vi "Server Create Event.vi"(8 "error in":errorcluster, 11 "server event ref":refnum<vi>) -> (0 "error out":errorcluster, 3 "server command event":refnum<user-event>)   [LabVIEW 2013]
doc: "Create user event for server operation commands."
uses:
  Server Event Start.ctl
  measure/Meas Sampling Configuration.ctl
  adc/ADC Trig Config.ctl
  adc/ADC Trig Mode Source.ctl
  adc/ADC Trig Coupling.ctl
  adc/ADC Trig Slope.ctl
  measure/processing/QWTB/Meas Proc QWTB Algorithm Parameter Data.ctl
  measure/processing/Meas Process Mode.ctl
  measure/processing/Meas Process Config.ctl
  measure/processing/Meas Process Raw Config.ctl
  measure/processing/Meas Process Raw Result Mode.ctl
  measure/processing/QWTB/Meas Proc QWTB Setup.ctl
  measure/processing/QWTB/Meas Proc QWTB Uncertainty Mode.ctl
  Server Event GUI command.ctl
  Server Event Command.ctl
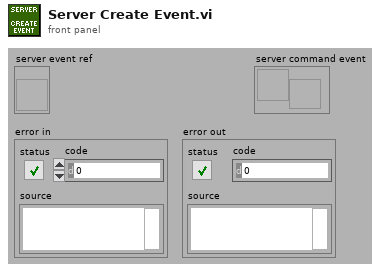
[diagram p1: front panel]
types:
  T1 = typedef "Server Event Start.ctl" = cluster{"client request":cluster{"meas config":T2, "mode":T8, "processing setup":T9}, "GUI request":T14, "command":T15}
  T2 = typedef "Meas Sampling Configuration.ctl" = cluster{"fs [Hz]":dbl, "count [smpl]":i64, "aperture [s]":dbl, "trigger":T3, "ranges [Vpk]":dbl[], "QWTB parameters":T7[]}
  T3 = typedef "ADC Trig Config.ctl" = cluster{"source":T4, "level [V]":dbl, "coupling":T5, "slope":T6}
  T4 = typedef "ADC Trig Mode Source.ctl" = enum16{"Immediate", "External", "Level"}
  T5 = typedef "ADC Trig Coupling.ctl" = enum16{"DC", "AC"}
  T6 = typedef "ADC Trig Slope.ctl" = enum16{"POS", "NEG"}
  T7 = typedef "Meas Proc QWTB Algorithm Parameter Data.ctl" = cluster{"name":string, "numerics":dbl[], "strings":string[]}
  T8 = typedef "Meas Process Mode.ctl" = enum16{"Raw", "QWTB"}
  T9 = typedef "Meas Process Config.ctl" = cluster{"mode":T8, "call after avgs?":bool, "calculate?":bool, "raw mode":T10, "QWTB":T12}
  T10 = typedef "Meas Process Raw Config.ctl" = cluster{"command":string, "result mode":T11, "res variable":string}
  T11 = typedef "Meas Process Raw Result Mode.ctl" = enum16{"Display console output (only Octave)", "Display string variable", "Display result file %respath%"}
  T12 = typedef "Meas Proc QWTB Setup.ctl" = cluster{"QWTB path":path, "alg filter path":string, "alg ids":string[], "alg parameters":string[], "parsed parameters":T7[], "selected alg":i32, "selected unc mode":T13, "qwtb mcc":i32, "qwtb timeout":i32, "qwtb covg":dbl}
  T13 = typedef "Meas Proc QWTB Uncertainty Mode.ctl" = enum16{"None", "GUF", "Monte Carlo"}
  T14 = typedef "Server Event GUI command.ctl" = cluster{"start":bool, "setup":bool, "setup&start":bool}
  T15 = typedef "Server Event Command.ctl" = enum16{"Identify", "Start", "Get status", "Get result"}
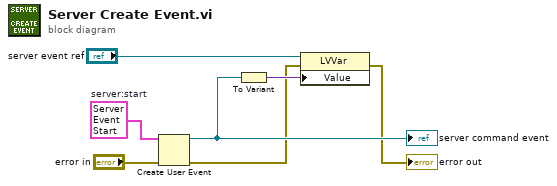
[diagram p0: block diagram]
diagram:
  w7 = T1 {"client request"={"meas config"={"fs [Hz]"=0.0, "count [smpl]"=0, "aperture [s]"=0.0, "trigger"={"source"=enum."Immediate", "level [V]"=0.0, "coupling"=enum."DC", "slope"=enum."POS"}, "ranges [Vpk]"=[], "QWTB parameters"=[]}, "mode"=enum."Raw", "processing setup"={"mode"=enum."Raw", "call after avgs?"=FALSE, "calculate?"=FALSE, "raw mode"={"command"="", "result mode"=enum."Display console output (only Octave)", "res variable"=""}, "QWTB"={"QWTB path"=path "", "alg filter path"="", "alg ids"=[], "alg parameters"=[], "parsed parameters"=[], "selected alg"=0, "selected unc mode"=enum."None", "qwtb mcc"=100, "qwtb timeout"=90, "qwtb covg"=95.0}}}, "GUI request"={"start"=FALSE, "setup"=FALSE, "setup&start"=FALSE}, "command"=enum."Identify"}  # server:start
  n1 = Create User Event(user event datatype=w7, error in="error in") -> (user event=w5:refnum<user-event>, error out=w1:errorcluster)
  "server command event" <- w5
  n2 = To Variant(anything=w5) -> (Variant=w2:variant)
  n3 = property class="LVVar"(reference="server event ref", error in=w1, "Value"=w2) -> (error out=→"error out":errorcluster)  [unwired: 1 out]
